vi "VernierHist.vi"(10 "Vernier Data":u16[](array[numeric]), 11 "Hist in":u16[][](array[numeric])) -> (3 "Hist out":u16[][](array[numeric]))   [LabVIEW 2014]
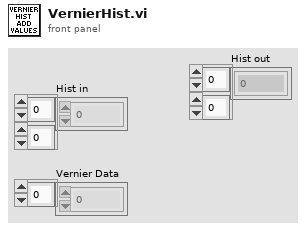
[diagram p1: front panel]
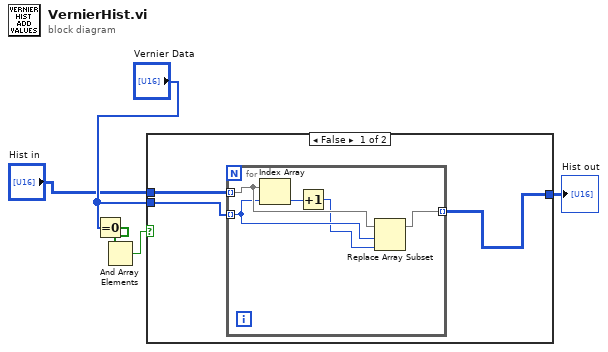
[diagram p0: block diagram]
diagram:
  n1 = Equal To 0?(x="Vernier Data") -> (x = 0?=w4:bool[])
  n2 = And Array Elements(Boolean array=w4) -> (logical AND=w3:bool)
  n3 = case shown="False" w3 {
    tunnel: "Vernier Data" -> [w8 _]
    tunnel: "Hist in" -> [w7 w14]
    tunnel: [w6 w14] -> w1
    frame False {
      n4 = for {
        tunnel: w7 -> [w12] mode=indexing
        tunnel: w8 -> [w10] mode=indexing
        tunnel: [w11] -> w6 mode=indexing
        n5 = Index Array(array=w12, index=w10) -> (element=w13:u16)
        n6 = Increment(x=w13) -> (x+1=w9:u16)
        n7 = Replace Array Subset(array=w12, new element=w9, index=w10) -> (w11:u16[])
      }
    }
    frame True {
    }
  }
  "Hist out" <- w1
